vi "cgpa.vi"() -> ()   [LabVIEW 2014]
uses:
  <vilib>/Utility/file.llb/Write To Spreadsheet File (string).vi
panel:
  out "cgpa":dbl
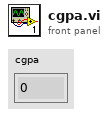
[diagram p1: front panel]
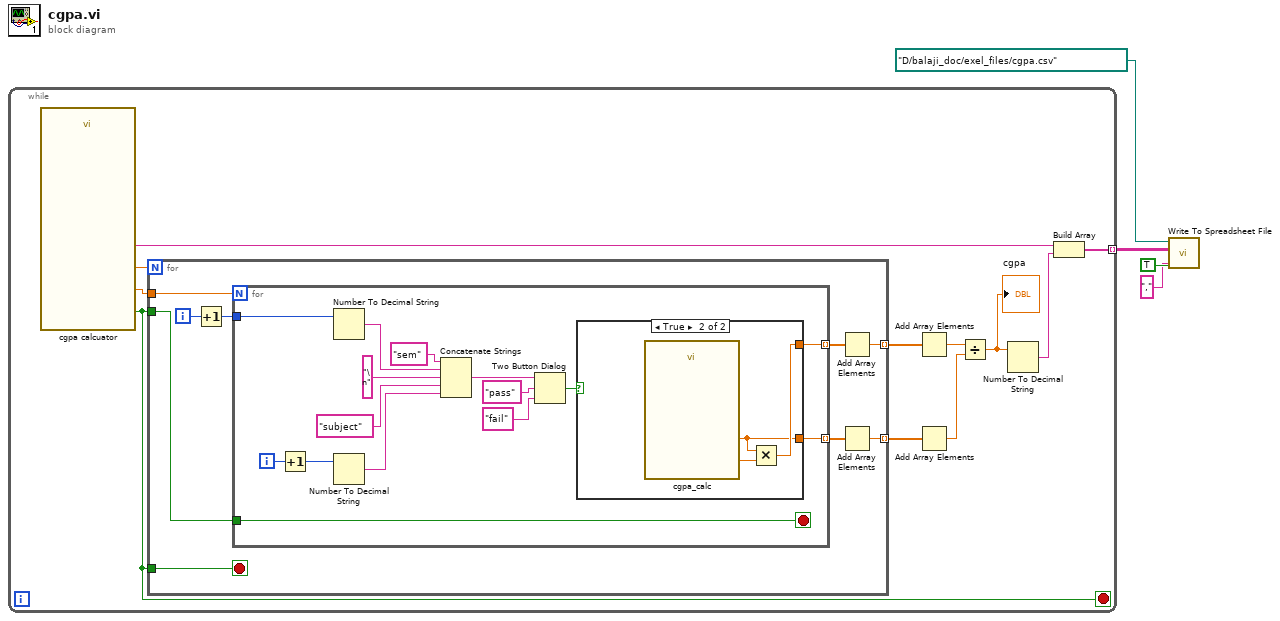
[diagram p0: block diagram]
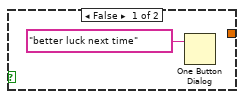
[diagram p2: hidden frame]
diagram:
  n1 = while {
    tunnel: [w6] -> w2 mode=indexing
    stop <- w5 stop-if-true
    n2 = call "cgpa calcuator"() -> ("end of students"=w5:bool, "number of subjects"=w15:dbl, "number of sems"=w14:dbl, "name of student"=w8:string)  [unwired: 14 in, 2 out]
    n3 = for {
      N: w14 -> [_]
      tunnel: w15 -> [w24]
      tunnel: [w20] -> w13 mode=indexing
      tunnel: [w18] -> w12 mode=indexing
      tunnel: w5 -> [w17]
      tunnel: w5 -> [w16]
      i -> [w23]
      stop <- w17 stop-if-true
      n4 = Increment(x=w23) -> (x+1=w22:i32)
      n5 = for {
        N: w24 -> [_]
        tunnel: w22 -> [w39]
        tunnel: [w27] -> w21 mode=indexing
        tunnel: [w26] -> w19 mode=indexing
        tunnel: w16 -> [w25]
        i -> [w38]
        stop <- w25 stop-if-true
        n6 = Increment(x=w38) -> (x+1=w37:i32)
        n7 = Number To Decimal String(number=w39) -> (decimal integer string=w35:string)  [unwired: 1 in]
        n8 = Number To Decimal String(number=w37) -> (decimal integer string=w32:string)  [unwired: 1 in]
        n9 = Concatenate Strings("sem", w35, "\n", "subject", w32) -> (w31:string)
        n10 = Two Button Dialog(message=w31, 1:"fail" ("F button name (\"Cancel\")"), 2:"pass" ("T button name (\"OK\")")) -> (T button?=w28:bool)
        n11 = case shown="True" w28 {
          tunnel: [_ w42] -> w27
          tunnel: [_ w41] -> w26
          frame False {
            n12 = One Button Dialog(message="better luck next time") -> ()  [unwired: 1 in, 1 out]
          }
          frame True {
            n13 = call "cgpa_calc"() -> ("marks"=w43:dbl, "grade points"=w41:dbl)  [unwired: 16 in, 2 out]
            n14 = Multiply(x=w41, y=w43) -> (x*y=w42:dbl)
          }
        }
      }
      n15 = Add Array Elements(numeric array=w21) -> (sum=w20:dbl)
      n16 = Add Array Elements(numeric array=w19) -> (sum=w18:dbl)
    }
    n17 = Add Array Elements(numeric array=w13) -> (sum=w11:dbl)
    n18 = Add Array Elements(numeric array=w12) -> (sum=w10:dbl)
    n19 = Divide(x=w11, y=w10) -> (x/y=w9:dbl)
    "cgpa" <- w9
    n20 = Number To Decimal String(number=w9) -> (decimal integer string=w7:string)  [unwired: 1 in]
    n21 = Build Array(w8, w7) -> (w6:string[])
  }
  n22 = call-poly <vilib>:"Write To Spreadsheet File.vi"("delimiter (\\t)"="," ("delimiter (\\t)"), "append to file? (new file:F)"=TRUE, "2D data"=w2, "file path (dialog if empty)"=path "D:/balaji_doc/exel_files/cgpa.csv") -> ()  [unwired: 4 in, 1 out]
